vi "Pathhorafech(SubVI)_varios.vi"(2 "error in":errorcluster, 3 "Folder path":path, 4 "Nº de acelerómetros":i32, 5 "Nº inductivos":i32) -> (0 "error out":errorcluster, 1 "Acel_Paths":path[](array[path]))   [LabVIEW 2015]
panel:
  out "date/time string":string
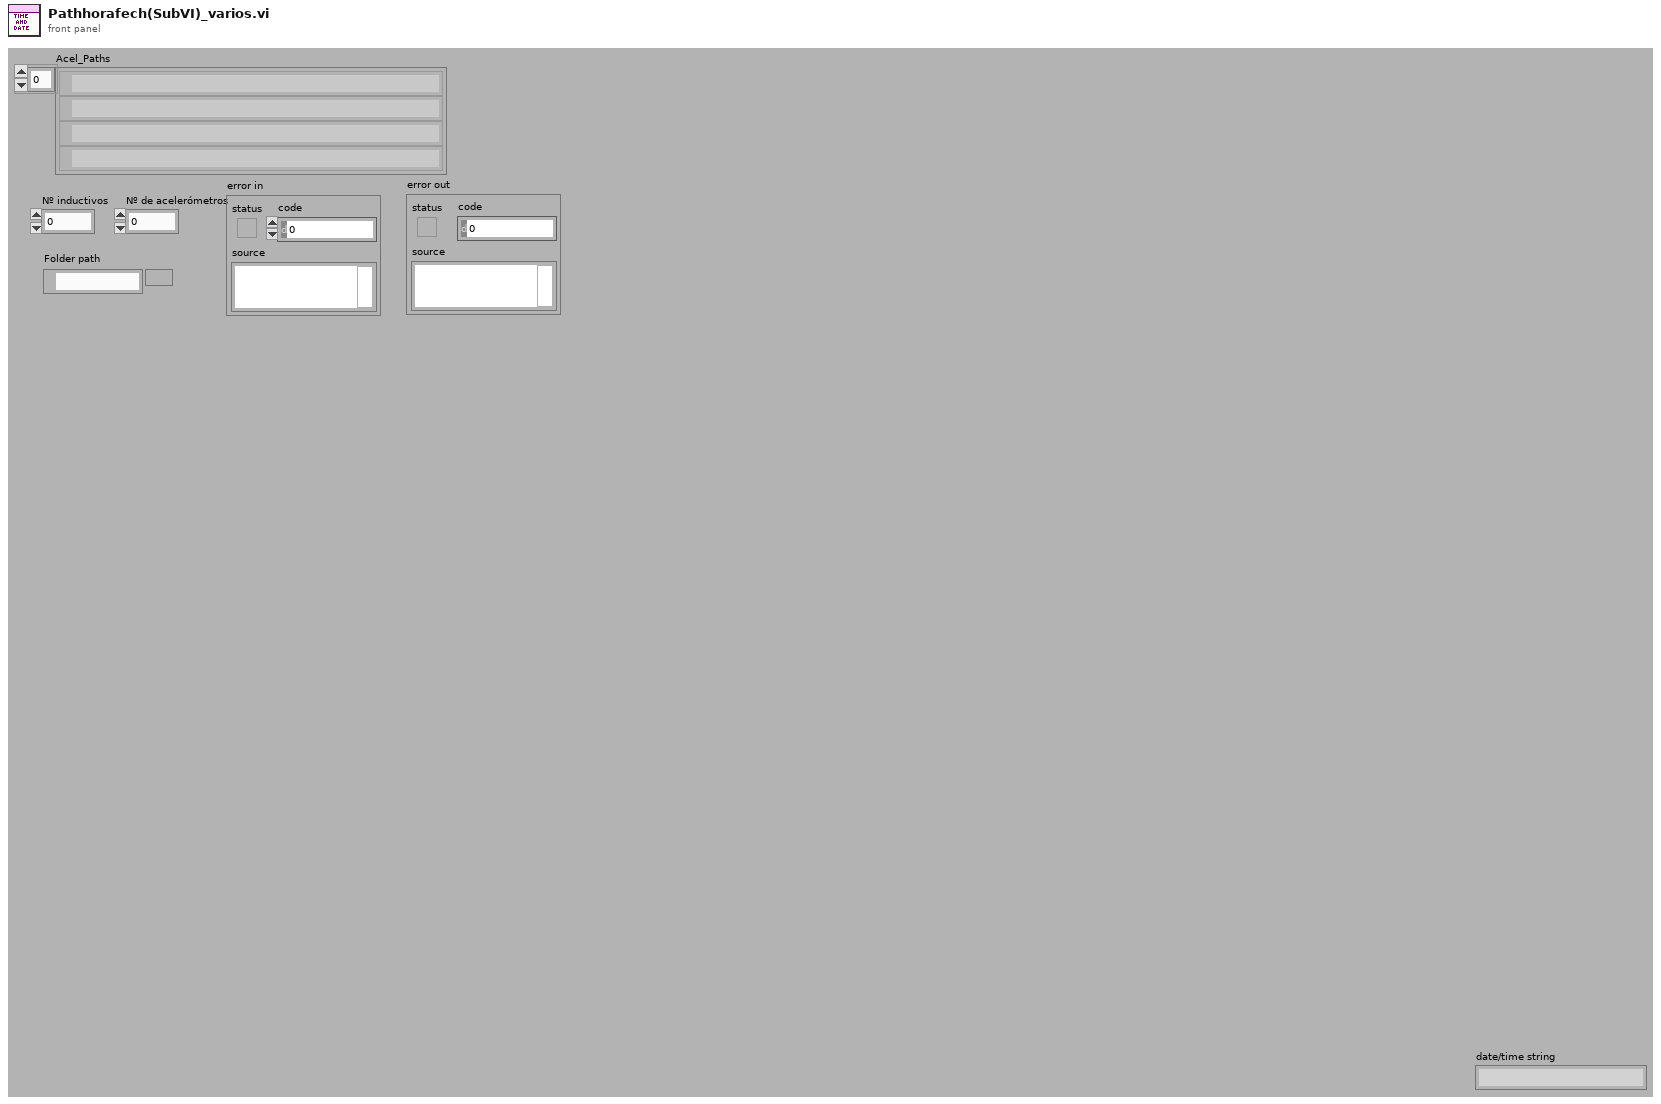
[diagram p1: front panel]
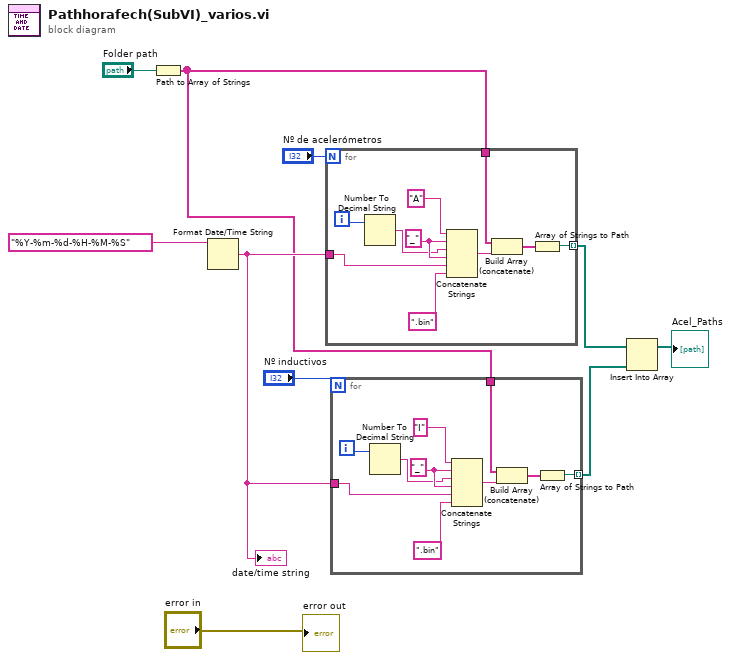
[diagram p0: block diagram]
diagram:
  n1 = Path to Array of Strings(0:"Folder path") -> (2:w5:string[])  [unwired: 1 out]
  n2 = Format Date/Time String(time format string (%c)="%Y-%m-%d-%H-%M-%S") -> (date/time string=w6:string)  [unwired: 2 in]
  "date/time string" <- w6
  n3 = for {
    N: "Nº de acelerómetros" -> [_]
    tunnel: w6 -> [w18]
    tunnel: w5 -> [w12]
    tunnel: [w11] -> w4 mode=indexing
    i -> [w19]
    w17 = "_" ("replace string (\"\")")
    n4 = Number To Decimal String(number=w19) -> (decimal integer string=w16:string)  [unwired: 1 in]
    n5 = Concatenate Strings("A" ("string"), w17, w16, w17, w18, ".bin" ("string")) -> (w13:string)
    n6 = Build Array (concatenate)(w12, w13) -> (w14:string[])
    n7 = Array of Strings to Path(0:w14) -> (2:w11:path)  [unwired: 1 out]
  }
  n8 = for {
    N: "Nº inductivos" -> [_]
    tunnel: w6 -> [w28]
    tunnel: w5 -> [w22]
    tunnel: [w21] -> w3 mode=indexing
    i -> [w29]
    w27 = "_" ("replace string (\"\")")
    n9 = Number To Decimal String(number=w29) -> (decimal integer string=w26:string)  [unwired: 1 in]
    n10 = Concatenate Strings("I" ("string"), w27, w26, w27, w28, ".bin" ("string")) -> (w23:string)
    n11 = Build Array (concatenate)(w22, w23) -> (w24:string[])
    n12 = Array of Strings to Path(0:w24) -> (2:w21:path)  [unwired: 1 out]
  }
  n13 = Insert Into Array(array=w4, new element=w3) -> (→"Acel_Paths":path[])  [unwired: 1 in]
  "error out" <- "error in"
